vi "TEST USER MANAGEMENT.vi"() -> ()   [LabVIEW 2009]
uses:
  User Access Type defs/All users access configuration cluster.ctl
  User Access Type defs/User access cluster array.ctl
  User Access Type defs/User access cluster.ctl
  User Access Type defs/Security level U8.ctl
panel:
  out "Access Configuration":T1 {"User array"."Expire sec" format="%.2f"}
  out "Valid user loged in?":bool
  out "User ID":string
  out "error in (no error)":errorcluster
  in  "Account Management":bool
  in  "Logout":bool
  in  "login":bool
  in  "stop":bool
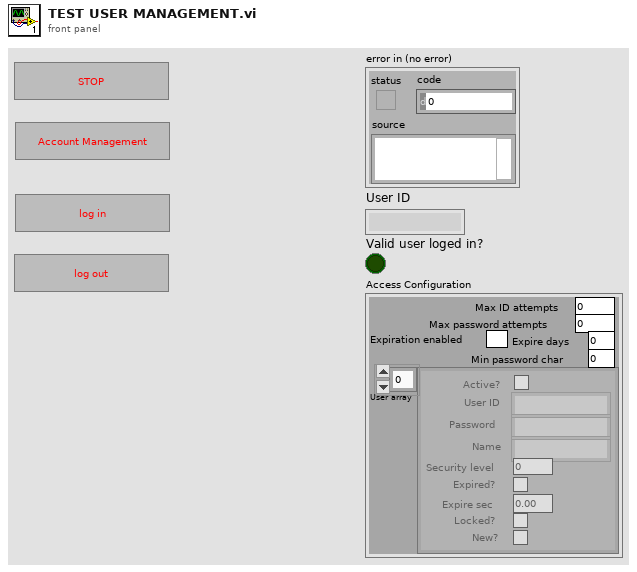
[diagram p1: front panel]
types:
  T1 = typedef "All users access configuration cluster.ctl" = cluster{"Max ID attempts":i32, "Max password attempts":i32, "Expiration enabled":bool, "Expire days":i32, "User array":T2, "Min password char":i32}
  T2 = typedef "User access cluster array.ctl" = T3[]
  T3 = typedef "User access cluster.ctl" = cluster{"Active?":bool, "User ID":string, "Password":string, "Name":string, "Security level":T4, "Expired?":bool, "Expire sec":dbl, "Locked?":bool, "New?":bool}
  T4 = typedef "Security level U8.ctl" = u8
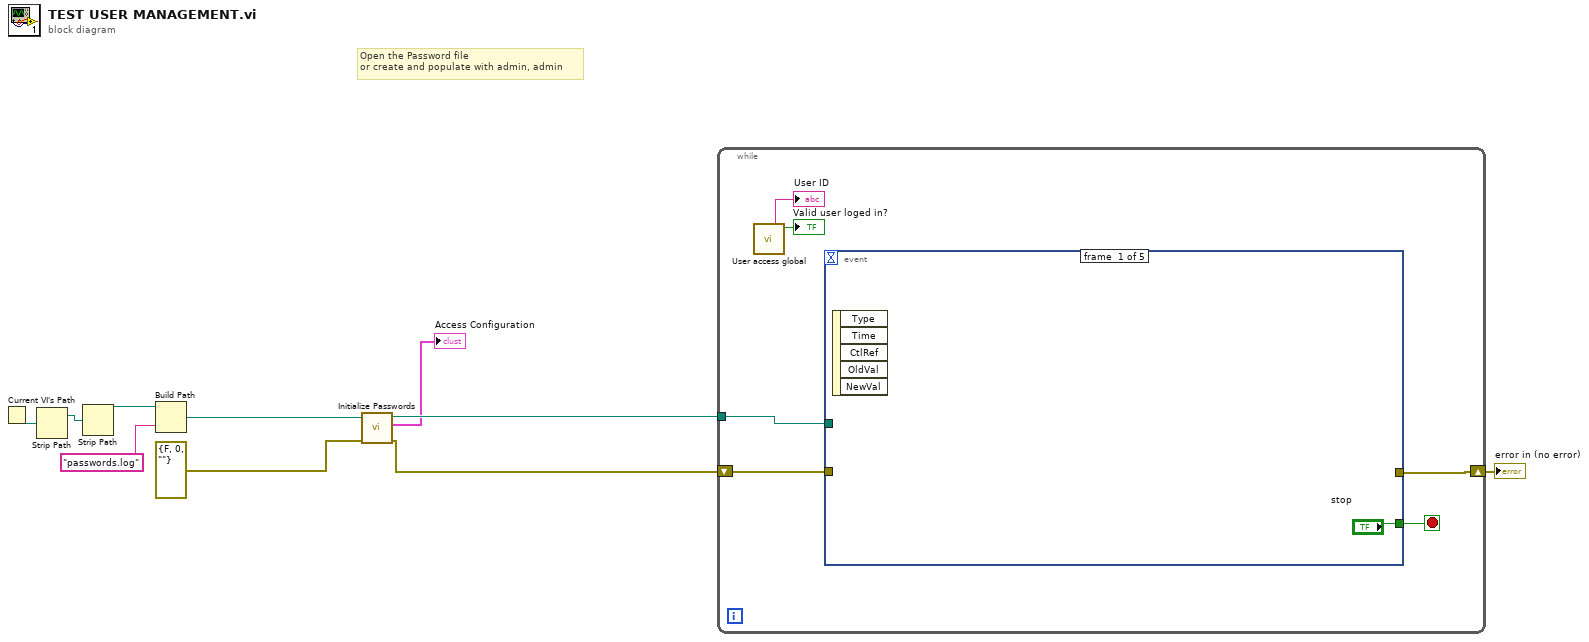
[diagram p0: block diagram]
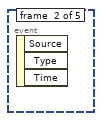
[diagram p2: hidden frame]
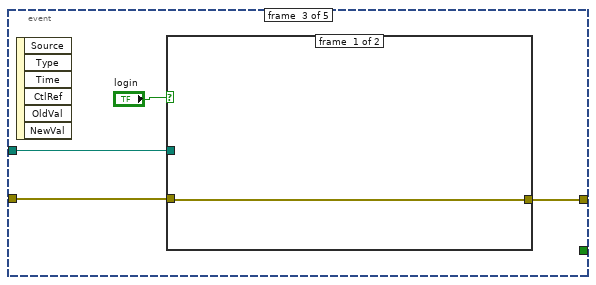
[diagram p3: hidden frame]
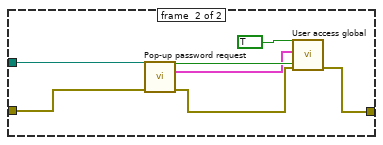
[diagram p4: hidden frame]
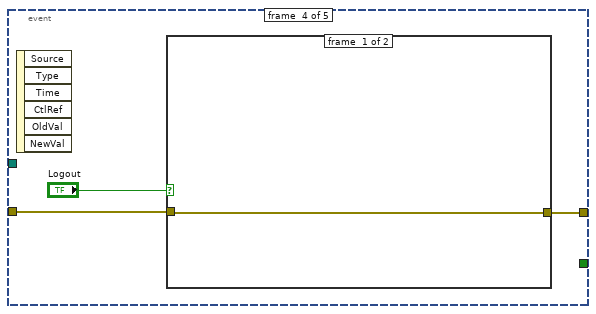
[diagram p5: hidden frame]
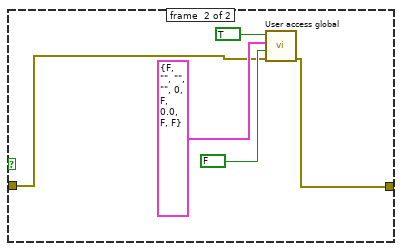
[diagram p6: hidden frame]
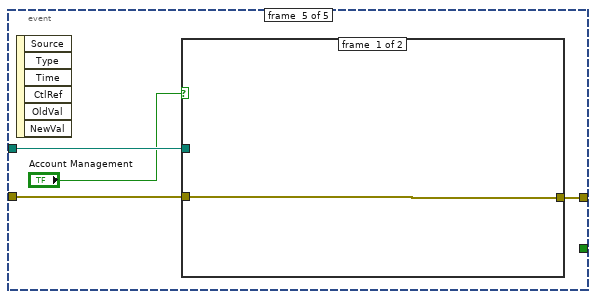
[diagram p7: hidden frame]
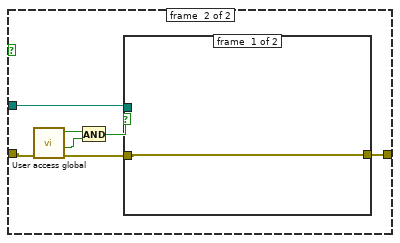
[diagram p8: hidden frame]
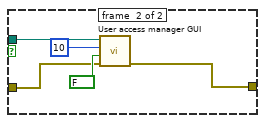
[diagram p9: hidden frame]
diagram:
  # "Open the Password file\nor create and populate with admin, admin"
  n1 = Current VI's Path() -> (path=w10:path)
  n2 = Strip Path(path=w10) -> (stripped path=w9:path)  [unwired: 1 out]
  n3 = Strip Path(path=w9) -> (stripped path=w8:path)  [unwired: 1 out]
  n4 = Build Path(base path=w8, name or relative path="passwords.log") -> (appended path=w5:path)
  n5 = call "Initialize Passwords.vi"("error in (no error)"=errorcluster {"status"=FALSE, "code"=0, "source"=""}, "Base path"=w5) -> ("error out"=w2:errorcluster, "Access Configuration"=→"Access Configuration":T1, "dup path"=w3:path)  [unwired: 7 out]
  n6 = while {
    shift-right: [w13] -> w6
    shift-left: w2 -> [w14]
    tunnel: w3 -> [w15]
    stop <- w16 stop-if-true
    n7 = call "User access global.vi"() -> ("Valid user loged in?"=→"Valid user loged in?":bool, "User ID"=→"User ID":string)  [unwired: 4 in, 6 out]
    n8 = event shown="[4] \"Account Management\": Value Change" {
      selector: _ -> [_ _ _ _ _]
      dyn-events: _ -> [_ _ _ _ _]
      timeout: _ -> [_ _ _ _ _]
      tunnel: ["stop" _ _ _ _] -> w16
      tunnel: w15 -> [_ _ w21 _ w42]
      tunnel: w14 -> [_ _ w20 w32 w41]
      tunnel: [_ _ w19 w31 w40] -> w13
      event #0 {
        n9 = event-data() -> ()  [unwired: 6 out]
      }
      event #1 {
        n10 = event-data() -> ()  [unwired: 4 out]
      }
      event #2 {
        n11 = event-data() -> ()  [unwired: 7 out]
        n12 = case shown="True" "login" {
          tunnel: w21 -> [_ w29]
          tunnel: w20 -> [w22 w28]
          tunnel: [w22 w23] -> w19
          frame #0 {
          }
          frame #1 {
            n13 = call "Pop-up password request.vi"("error in (no error)"=w28, "Filepath"=w29) -> ("error out"=w24:errorcluster, "User access cluster"=w25:T3, "Valid password?"=w27:bool)  [unwired: 3 out]
            n14 = call "User access global.vi"("error in (no error)"=w24, "Set Loged in"=w27, "User access set"=w25, "Set? (get)"=TRUE) -> ("error out"=w23:errorcluster)  [unwired: 7 out]
          }
        }
      }
      event #3 {
        n15 = event-data() -> ()  [unwired: 7 out]
        n16 = case shown="True" "Logout" {
          tunnel: w32 -> [w33 w35]
          tunnel: [w33 w34] -> w31
          frame #0 {
          }
          frame #1 {
            n17 = call "User access global.vi"("error in (no error)"=w35, "Set Loged in"=FALSE, "User access set"=T3 {"Active?"=FALSE, "User ID"="", "Password"="", "Name"="", "Security level"=0, "Expired?"=FALSE, "Expire sec"=0.0, "Locked?"=FALSE, "New?"=FALSE}, "Set? (get)"=TRUE) -> ("error out"=w34:errorcluster)  [unwired: 7 out]
          }
        }
      }
      event #4 {
        n18 = event-data() -> ()  [unwired: 7 out]
        n19 = case shown="True" "Account Management" {
          tunnel: w42 -> [_ w50]
          tunnel: w41 -> [w43 w48]
          tunnel: [w43 w49] -> w40
          frame #0 {
          }
          frame #1 {
            n20 = call "User access global.vi"("error in (no error)"=w48) -> ("error out"=w47:errorcluster, "Administrator"=w45:bool, "Valid user loged in?"=w46:bool)  [unwired: 3 in, 5 out]
            n21 = And(x=w46, y=w45) -> (x .and. y?=w44:bool)
            n22 = case shown="True" w44 {
              tunnel: w50 -> [_ w54]
              tunnel: [w51 w53] -> w49
              tunnel: w47 -> [w51 w52]
              frame #0 {
              }
              frame #1 {
                n23 = call "User access manager GUI.vi"("error in (no error)"=w52, "Part 11?"=FALSE, "Security level"=T4 10, "Password Filepath"=w54) -> ("error out"=w53:errorcluster)  [unwired: 7 out]
              }
            }
          }
        }
      }
    }
  }
  "error in (no error)" <- w6
